vi "Error Query.vi"(8 "error in (no error)":errorcluster, 11 "VISA resource name":refnum<visa-resource-name>) -> (0 "error out":errorcluster, 1 "Error Message":string, 2 "Error Code":i32[](array[numeric]), 3 "VISA resource name out":refnum<visa-resource-name>)   [LabVIEW 2015, in "Tektronix DPO MSO 2000 4000 Series.lvlib"]
doc: "Queries an instrument for any errors in the error queue of the instrument. The Error Query VI continuously reads errors until this VI reads all the errors from the instrument. \n<B>Note</B>: Because most driver VIs automatically call the Error Query VI, you do not need to call this VI in an application."
uses:
  Tektronix DPO MSO 2000 4000 Series.lvlib
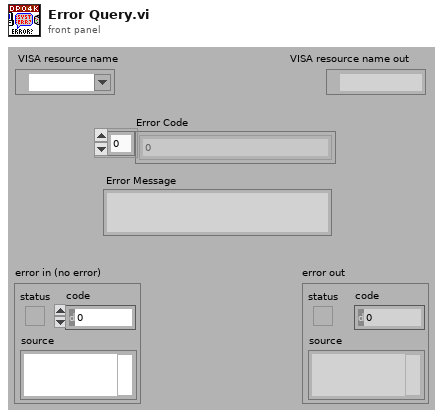
[diagram p1: front panel]
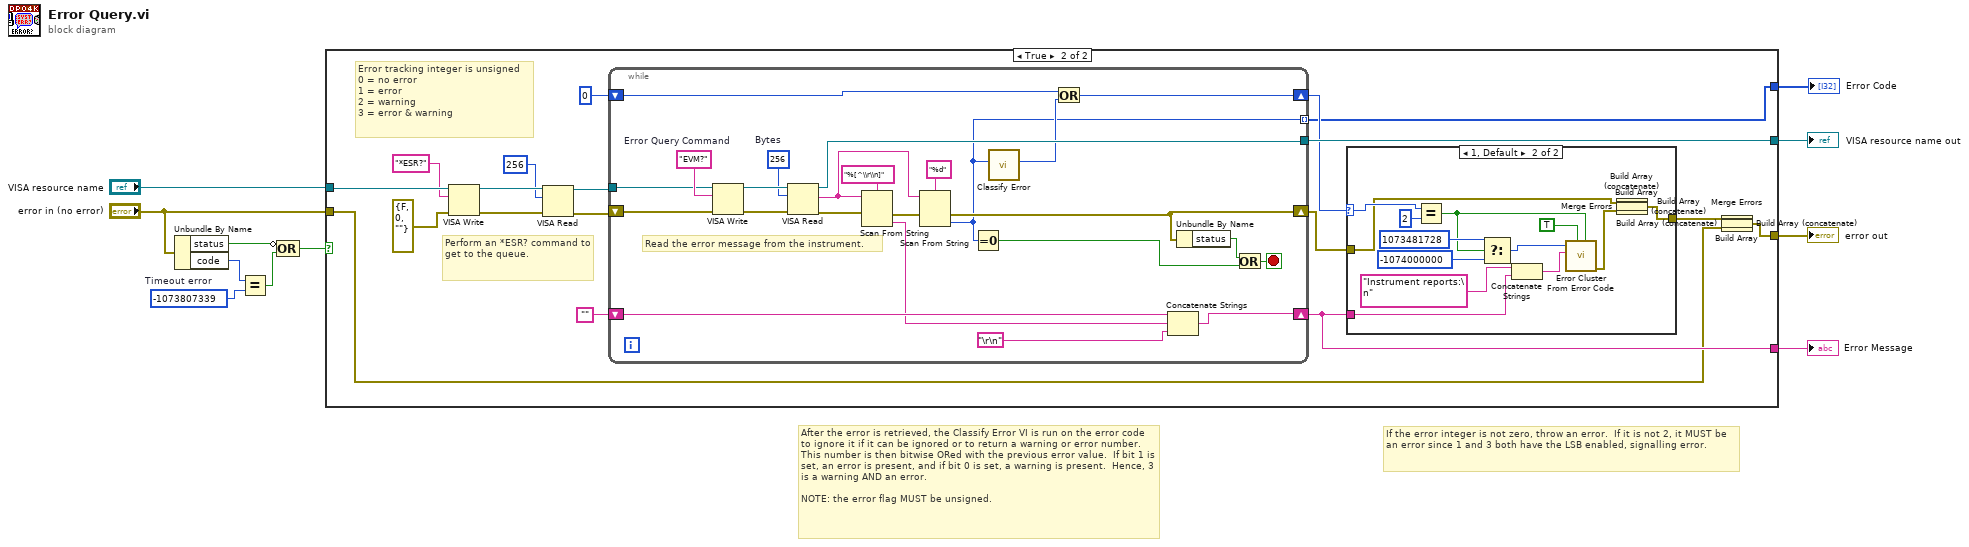
[diagram p0: block diagram]
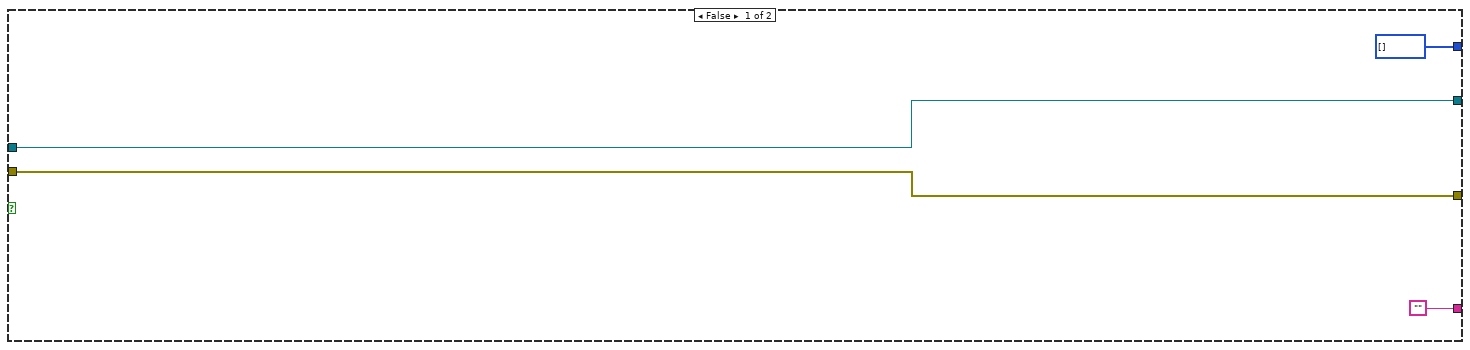
[diagram p2: hidden frame]
diagram:
  w6 = -1073807339  # Timeout error
  # "If the error integer is not zero, throw an error.  If it is not 2, it MUST be an error since 1 and 3 both have the LSB enabled, signalling error."
  # "After the error is retrieved, the Classify Error VI is run on the error code to ignore it if it can be ignored or to return a warning or error number.  This number is then bitwise ORed with the previous error value.  If bit 1 is set, an error is present, and if bit 0 is set, a warning is present.  Hence, 3 is a warning AND an error.\n\nNOTE: the error flag MUST be unsigned."
  n1 = Unbundle By Name("error in (no error)") -> ("status"=w7:bool, "code"=w4:i32)
  n2 = Equal?(x=w4, y=w6) -> (x = y?=w5:bool)
  n3 = Compound Arithmetic op=OR(invert w7, w5) -> (w3:bool)
  n4 = case shown="True" w3 {
    tunnel: [w15 w36] -> w11
    tunnel: "VISA resource name" -> [w15 w32]
    tunnel: "error in (no error)" -> [w14 w19]
    tunnel: [w14 w34] -> w9
    tunnel: ["" w33] -> w2
    tunnel: [i32[] [] w21] -> w1
    frame False {
    }
    frame True {
      # "Error tracking integer is unsigned\n0 = no error\n1 = error\n2 = warning\n3 = error & warning"
      # "Perform an *ESR? command to get to the queue."
      n5 = VISA Write(VISA resource name=w32, write buffer="*ESR?", error in (no error)=errorcluster {"status"=FALSE, "code"=0, "source"=""}) -> (VISA resource name out=w29:refnum<visa-resource-name>, error out=w30:errorcluster)  [unwired: 1 out]
      n6 = VISA Read(VISA resource name=w29, byte count=u32 256, error in (no error)=w30) -> (VISA resource name out=w27:refnum<visa-resource-name>, error out=w26:errorcluster)  [unwired: 2 out]
      n7 = while {
        tunnel: [w77] -> w36
        tunnel: w27 -> [w60]
        shift-right: [w66] -> w33
        shift-left: "" -> [w68]
        shift-right: [w57] -> w24
        shift-left: u32 0 ("x = 0?") -> [w56]
        shift-right: [w64] -> w23
        shift-left: w26 -> [w65]
        tunnel: [w54] -> w21 mode=indexing
        stop <- w71 stop-if-true
        w75 = u32 256  # Bytes
        w73 = "EVM?"  # Error Query Command
        # "Read the error message from the instrument."
        n8 = VISA Write(VISA resource name=w60, write buffer=w73, error in (no error)=w65) -> (VISA resource name out=w76:refnum<visa-resource-name>, error out=w74:errorcluster)  [unwired: 1 out]
        n9 = VISA Read(VISA resource name=w76, byte count=w75, error in (no error)=w74) -> (VISA resource name out=w77:refnum<visa-resource-name>, read buffer=w69:string, error out=w63:errorcluster)  [unwired: 1 out]
        n10 = Scan From String(format string="%[^\\r\\n]", input string=w69, error in=w63) -> (error out=w62:errorcluster, output 1=w67:string)  [unwired: 2 in, 2 out]
        n11 = Scan From String(format string="%d", input string=w69, error in=w62) -> (error out=w64:errorcluster, output 1=w54:i32)  [unwired: 2 in, 2 out]
        n12 = Equal To 0?(x=w54) -> (x = 0?=w59:bool)
        n13 = call "Classify Error.vi"("Error Code"=w54) -> ("Error Classification"=w55:i32)  [unwired: 10 in]
        n14 = Or(x=w56, y=w55) -> (x .or. y?=w57:u32)
        n15 = Concatenate Strings(w68, w67, "\r\n") -> (w66:string)
        n16 = Unbundle By Name(w64) -> ("status"=w61:bool)
        n17 = Or(x=w61, y=w59) -> (x .or. y?=w71:bool)
      }
      n18 = case shown="1, Default" w24 {
        selector: w24 -> [_ w49]
        tunnel: [w37 w41] -> w20
        tunnel: w33 -> [_ w50]
        tunnel: w23 -> [w37 w43]
        frame 0 {
        }
        frame 1, Default {
          n19 = Equal?(x=w49, y=u32 2) -> (x = y?=w46:bool)
          n20 = Select(t=1073481728 ("Code"), s=w46, f=-1074000000 ("Code")) -> (s? t:f=w44:i32)
          n21 = Concatenate Strings("Instrument reports:\n" ("Source"), w50) -> (w51:string)
          n22 = call <vilib>:"Error Cluster From Error Code.vi"("is warning? (False)"=w46, "show call chain? (False)"=TRUE, "error message (\"\")"=w51, "error code (0)"=w44) -> ("error out"=w42:errorcluster)  [unwired: 5 in]
          n23 = Build Array(w43, w42) -> (w40:errorcluster[])
          n24 = Build Array (concatenate)(w40) -> (w39:errorcluster[])
          n25 = Build Array (concatenate)(w39) -> (w38:errorcluster[])
          n26 = Merge Errors(w38) -> (w41:errorcluster)
        }
      }
      n27 = Build Array(w20, w19) -> (w18:errorcluster[])
      n28 = Build Array (concatenate)(w18) -> (w17:errorcluster[])
      n29 = Build Array (concatenate)(w17) -> (w16:errorcluster[])
      n30 = Merge Errors(w16) -> (w34:errorcluster)
    }
  }
  "VISA resource name out" <- w11
  "error out" <- w9
  "Error Message" <- w2
  "Error Code" <- w1
